vi "ReconnectProcedureScalar.vi"(2 "Error In":errorcluster, 3 "Port Number":u16, 4 "TCP In":refnum<k5>) -> (0 "Error Out":errorcluster, 1 "TCP Out":refnum<k5>)   [LabVIEW 2014]
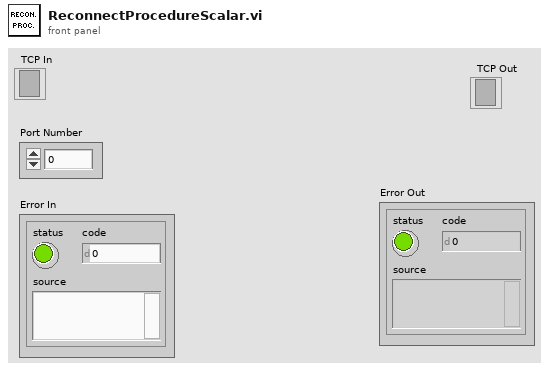
[diagram p1: front panel]
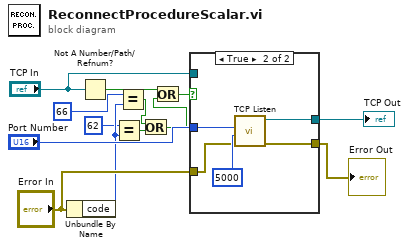
[diagram p0: block diagram]
diagram:
  n1 = Unbundle By Name("Error In") -> ("code"=w5:i32)
  n2 = Not A Number/Path/Refnum?(number/path/refnum="TCP In") -> (NaN/Path/Refnum?=w12:bool)
  n3 = Equal?(x=62, y=w5) -> (x = y?=w3:bool)
  n4 = Equal?(x=66, y=w5) -> (x = y?=w2:bool)
  n5 = Or(x=w2, y=w3) -> (x .or. y?=w1:bool)
  n6 = Or(x=w12, y=w1) -> (x .or. y?=w10:bool)
  n7 = case shown="True" w10 {
    tunnel: "TCP In" -> [w15 _]
    tunnel: "Error In" -> [w14 w16]
    tunnel: "Port Number" -> [_ w20]
    tunnel: [w14 w19] -> w6
    tunnel: [w15 w18] -> w7
    frame False {
    }
    frame True {
      n8 = call <vilib>:"TCP Listen.vi"("error in (no error)"=w16, "timeout ms (wait forever: -1)"=5000, "port"=w20) -> ("error out"=w19:errorcluster, "connection ID"=w18:refnum<k5>)  [unwired: 4 in, 3 out]
    }
  }
  "TCP Out" <- w7
  "Error Out" <- w6
